vi "test U16-2.vi"(11 "Test Case In":refnum<class "Build Sequence Test.lvclass">) -> (0 "error out":errorcluster, 3 "Test Case Out":refnum<class "Build Sequence Test.lvclass">)   [LabVIEW 2020, in "Build Sequence Test.lvclass"]
uses:
  Tests/SDO download U16 Test/Build Sequence Test.lvclass
  Tests/SDO download U16 Test/Build Sequence Test.lvclass/Build Sequence Test.ctl
  4993e8ee-a06a-463a-9684-69129f64d5ce.vi
  CANopen.lvclass
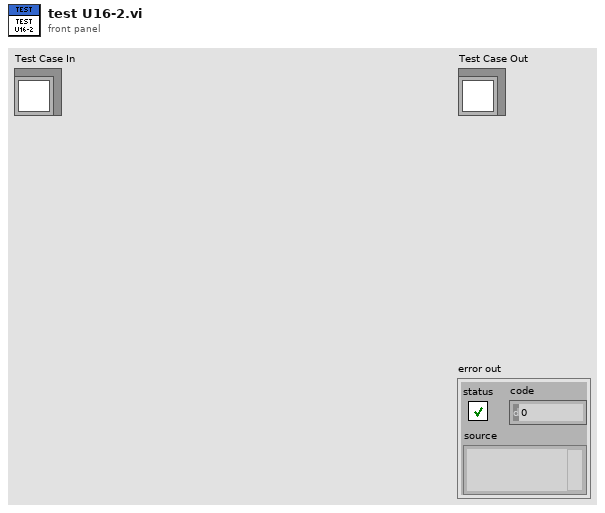
[diagram p1: front panel]
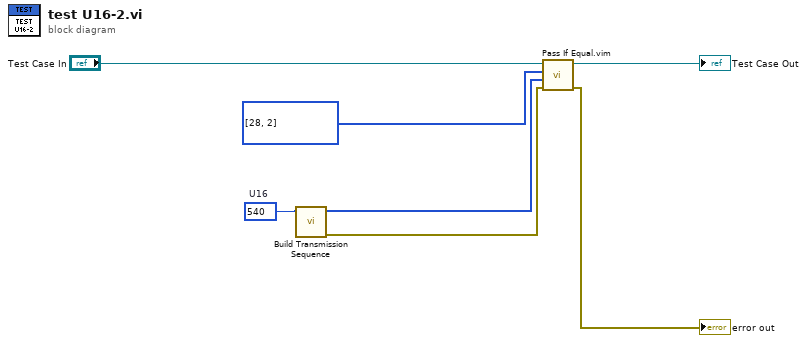
[diagram p0: block diagram]
diagram:
  w4 = u16 540  # U16
  n1 = call "Build Transmission Sequence.vi"("Data"=w4) -> ("error out"=w1:errorcluster, "Transmission Sequence"=w3:u8[])  [unwired: 9 in]
  n2 = call "Pass If Equal.vim"("error in (no error)"=w1, "Actual"=w3, "Expected"=u8[] [28, 2] ("appended array"), "LUnit Test Case In"="Test Case In") -> ("error out"=→"error out":errorcluster, "LUnit Test Case Out"=→"Test Case Out":refnum<class "Build Sequence Test.lvclass">)  [unwired: 6 in]
